vi "Read Read Only.vi"(8 "error in (no error)":errorcluster, 11 "Const_CPLX_EXT in":refnum<class "Const_CPLX_EXT.lvclass">) -> (0 "error out":errorcluster, 2 "Read Only":bool, 3 "Const_CPLX_EXT out":refnum<class "Const_CPLX_EXT.lvclass">)   [LabVIEW 2021, in "Const_CPLX_EXT.lvclass"]
uses:
  Const_CPLX_EXT.lvclass
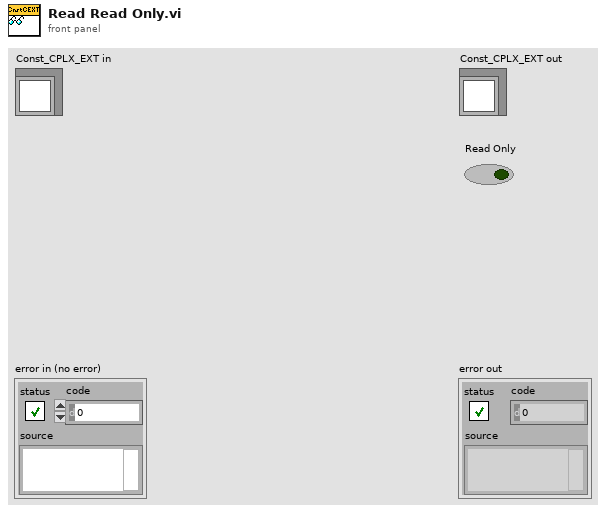
[diagram p1: front panel]
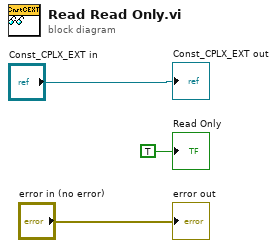
[diagram p0: block diagram]
diagram:
  "error out" <- "error in (no error)"
  "Const_CPLX_EXT out" <- "Const_CPLX_EXT in"
  "Read Only" <- TRUE ("Read Only")
